vi "Text Format Duration.vi"(8 "error in (no error)":errorcluster, 11 "Test Info in":refnum<class "Test Info.lvclass">) -> (0 "error out":errorcluster, 3 "Test Info out":refnum<class "Test Info.lvclass">)   [LabVIEW 2023, in "Data Analysis.lvlib" / "Test Info.lvlib" / "Test Info.lvclass"]
uses:
  Test Info.lvclass
panel:
  out "length":i32
  in  "String":string
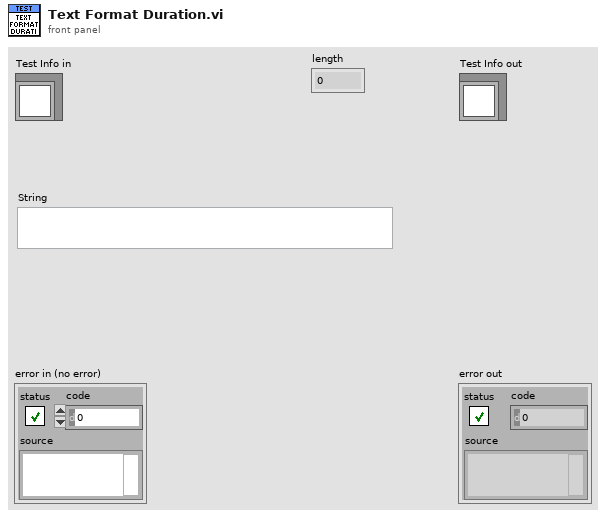
[diagram p1: front panel]
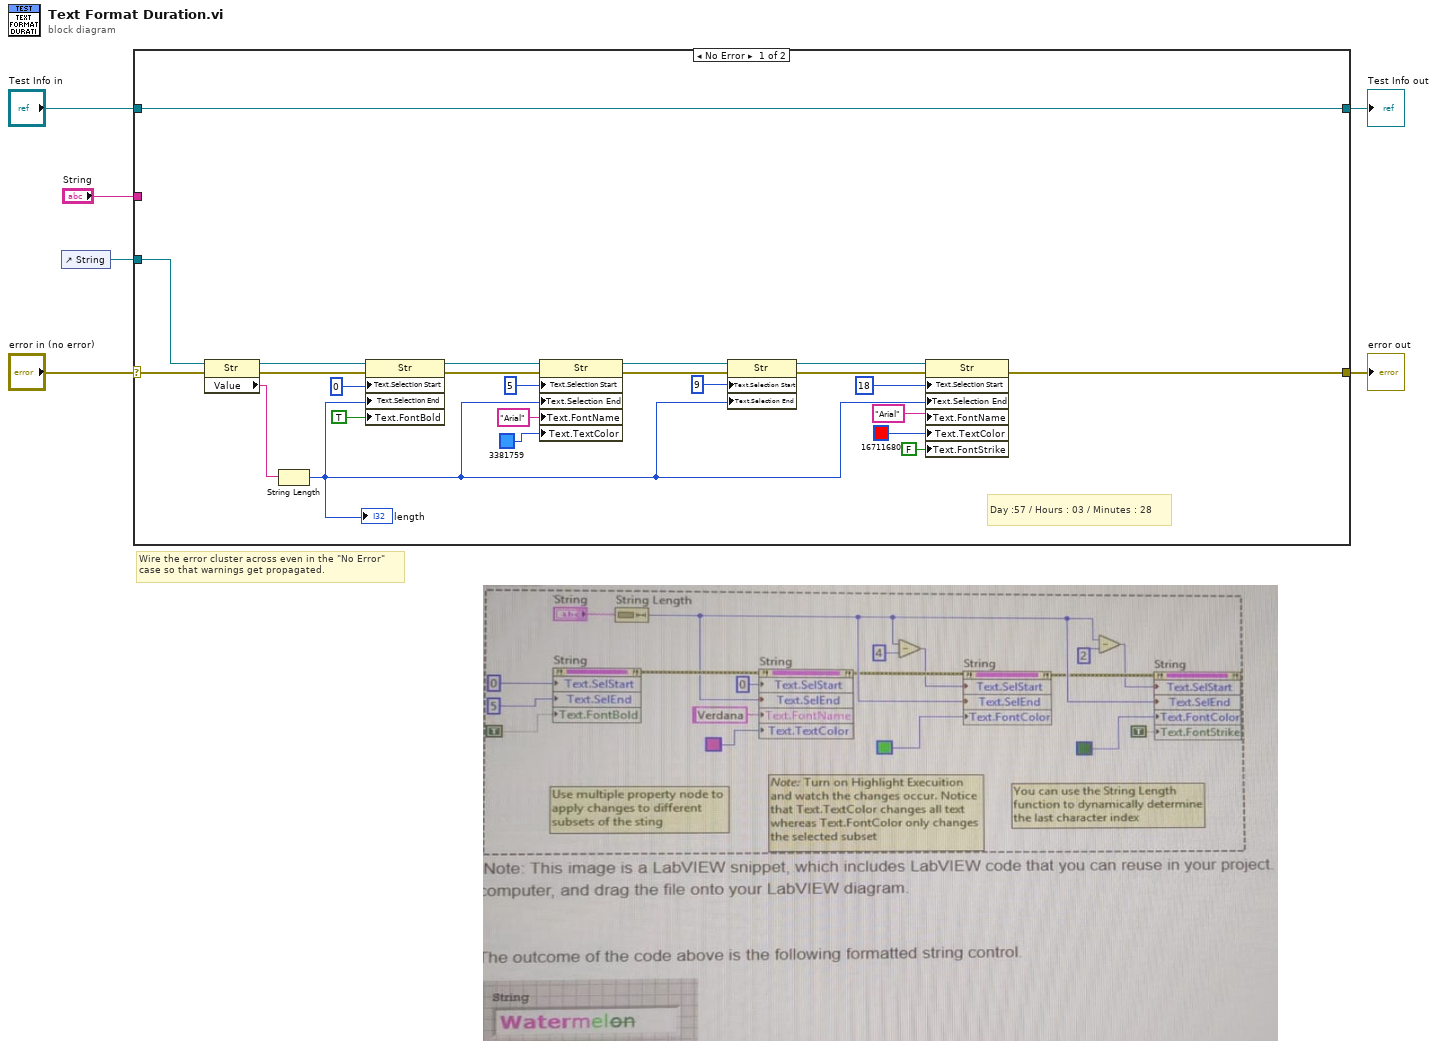
[diagram p0: block diagram]
diagram:
  # "Wire the error cluster across even in the \"No Error\"\ncase so that warnings get propagated."
  n1 = control-ref of="String"() -> (w1:refnum<vi>)
  n2 = case shown="No Error" "error in (no error)" {
    selector: "error in (no error)" -> [w11 w32]
    tunnel: [w15 w32] -> w5
    tunnel: [w30 w31] -> w3
    tunnel: "Test Info in" -> [w30 w31]
    tunnel: "String" -> [_ _]
    tunnel: w1 -> [w7 _]
    frame No Error {
      # "Day :57 / Hours : 03 / Minutes : 28"
      n3 = property class="Str"(reference=w7, error in=w11) -> (reference out=w9:refnum<vi>, error out=w10:errorcluster, "Value"=w8:string)
      n4 = String Length(string=w8) -> (length=w13:i32)
      "length" <- w13
      n5 = property class="Str"(reference=w9, error in=w10, "Text.Selection Start"=u32 0 ("Text.Selection:Start"), "Text.Selection End"=w13, "Text.FontBold"=TRUE ("Text.Font:Bold")) -> (reference out=w17:refnum<vi>, error out=w27:errorcluster)
      n6 = property class="Str"(reference=w17, error in=w27, "Text.Selection Start"=u32 5 ("Text.Selection:Start"), "Text.Selection End"=w13, "Text.FontName"="Arial" ("Text.Font:Name"), "Text.TextColor"=u32 3381759 ("Text.Text Colors:Text Color")) -> (reference out=w18:refnum<vi>, error out=w19:errorcluster)
      n7 = property class="Str"(reference=w18, error in=w19, "Text.Selection Start"=u32 9 ("Text.Selection:Start"), "Text.Selection End"=w13) -> (reference out=w16:refnum<vi>, error out=w22:errorcluster)
      n8 = property class="Str"(reference=w16, error in=w22, "Text.Selection Start"=u32 18 ("Text.Selection:Start"), "Text.Selection End"=w13, "Text.FontName"="Arial" ("Text.Font:Name"), "Text.TextColor"=u32 16711680 ("Text.Text Colors:Text Color"), "Text.FontStrike"=FALSE ("Text.Font:Strikeout")) -> (error out=w15:errorcluster)  [unwired: 1 out]
    }
    frame Error {
    }
  }
  "error out" <- w5
  "Test Info out" <- w3
